vi "Blinking LED WiringPi.so.vi"() -> ()   [LabVIEW 2014]
uses:
  WiringPi Pin Mode.ctl
  libwiringPi.so
panel:
  out "Status 3":bool
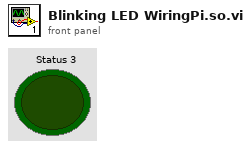
[diagram p1: front panel]
types:
  T1 = typedef "WiringPi Pin Mode.ctl" = enum8{"INPUT", "OUTPUT", "PWM_OUTPUT", "GPIO_CLOCK", "SOFT_PWM_OUTPUT", "SOFT_TONE_OUTPUT", "PWM_TONE_OUTPUT"}
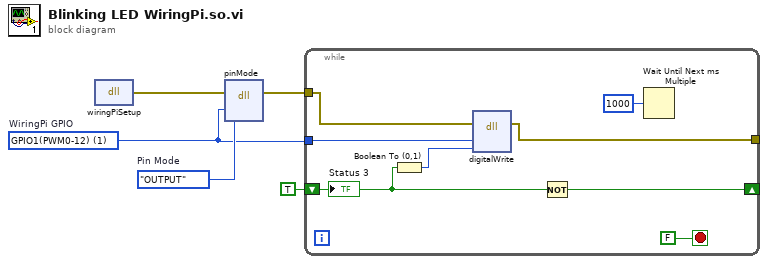
[diagram p0: block diagram]
diagram:
  w1 = u8 1 items=["SDA(I2C)-3"=8, "SCL(I2C)-5"=9, "MOSI(SPI)-19"=12, "MISO(SPI)-21"=13, "SCLK(SPI)-23"=14, "GPIO2-13"=2, "GPIO3-15"=3, "GPIO4-16"=4, "GPIO5-18"=5, "GPIO6-22"=6, "GPIO7-7"=7, "GPIO21-29"=21, "GPIO22-31"=22, "GPIO25-37"=25, "GPIO27-36"=27, "GPIO26(PWM0)-32"=26, "GPIO1(PWM0-12)"=1, "GPIO23(PWM1)-14"=23, "GPIO24(PWM1)-35"=24, "TXD(UART)-8"=15, "RXD(UART)-10"=16, "GPIO10(CE0-SPI)-24"=10, "GPPI11(CE1)-SPI)-26"=11, "GPIO28(PCM_DIN)36"=28, "GPIO29(PCM_DOUT)40"=29]  # WiringPi GPIO
  w3 = WiringPi_Pin_Mode."OUTPUT"  # Pin Mode
  n1 = dll-call lib="libwiringPi.so" fn="wiringPiSetup"() -> (error out=w4:errorcluster)  [unwired: 4 in, 1 out]
  n2 = dll-call lib="libwiringPi.so" fn="pinMode"(error in=w4, "pin"=w1, "state"=w3) -> (error out=w2:errorcluster)  [unwired: 5 in, 1 out]
  n3 = while {
    shift-right: [w11] -> _
    shift-left: TRUE -> [w8]
    tunnel: w2 -> [w10]
    tunnel: w1 -> [w9]
    tunnel: [w6] -> _
    stop <- FALSE stop-if-true
    n4 = Boolean To (0,1)(Boolean=w8) -> (0, 1=w7:i16)
    n5 = dll-call lib="libwiringPi.so" fn="digitalWrite"(error in=w10, "pin"=w9, "value"=w7) -> (error out=w6:errorcluster)  [unwired: 5 in, 1 out]
    n6 = Not(x=w8) -> (.not. x?=w11:bool)
    n7 = Wait Until Next ms Multiple(millisecond multiple=u32 1000) -> ()  [unwired: 1 out]
    "Status 3" <- w8
  }
